vi "Tote Barrel Array Test.vi"() -> ()   [LabVIEW 2014]
panel:
  in  "Release":bool
  in  "Height":dbl
  out "Array Index":dbl
  out "Array Output":dbl
  in  "Down Button":bool
  in  "Up Button":bool
  in  "Grab Barrel":bool
  in  "Grab Tote":bool
  out "Barrel Grab":bool
  out "Tote Grabbed":bool
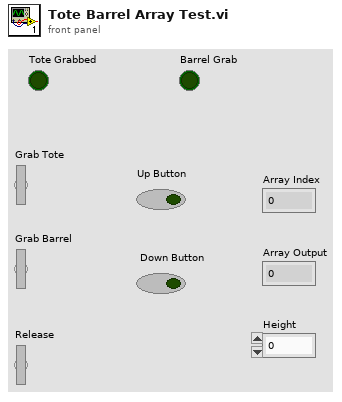
[diagram p1: front panel]
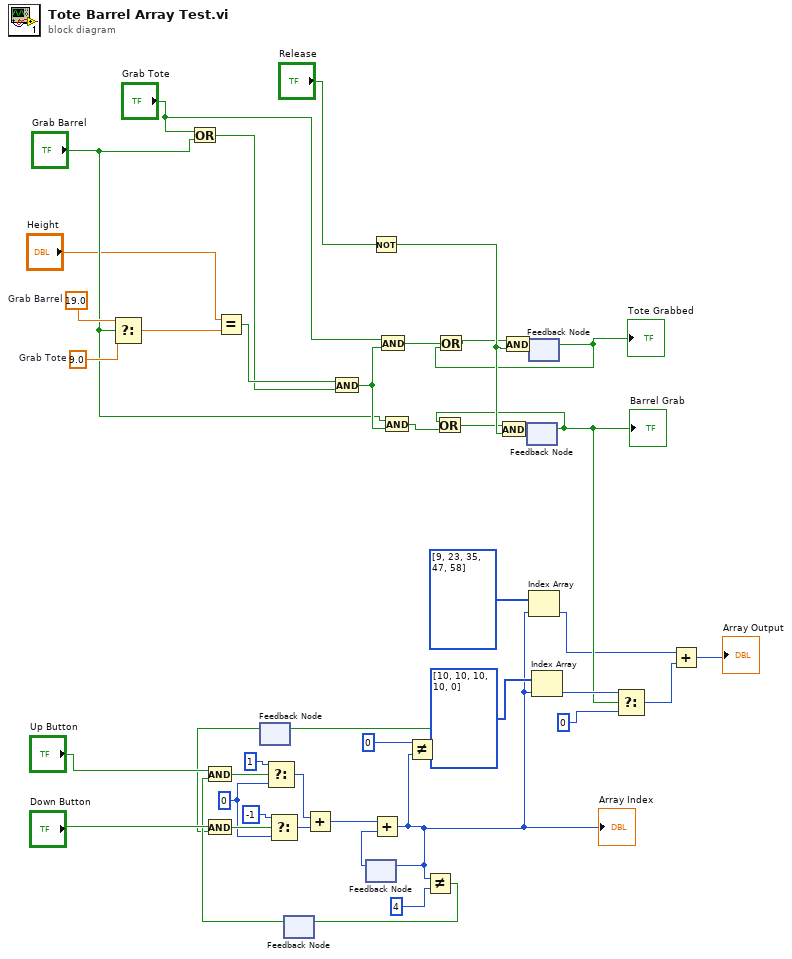
[diagram p0: block diagram]
diagram:
  w33 = 0
  w42 = 19.0  # Grab Barrel
  w43 = 9.0  # Grab Tote
  n1 = Select(t=w42, s="Grab Barrel", f=w43) -> (s? t:f=w41:dbl)
  n2 = Or(x="Grab Tote", y="Grab Barrel") -> (x .or. y?=w38:bool)
  n3 = Equal?(x="Height", y=w41) -> (x = y?=w44:bool)
  n4 = feedback #1() -> (w18:bool)  [unwired: 1 in]
  n5 = And(x="Down Button", y=w18) -> (x .and. y?=w37:bool)
  n6 = Select(t=-1, s=w37, f=w33) -> (s? t:f=w31:i32)
  n7 = feedback #2() -> (w21:bool)  [unwired: 1 in]
  n8 = And(x="Up Button", y=w21) -> (x .and. y?=w36:bool)
  n9 = Select(t=1, s=w36, f=w33) -> (s? t:f=w32:i32)
  n10 = Add(x=w32, y=w31) -> (x+y=w28:i32)
  n11 = And(x=w44, y=w38) -> (x .and. y?=w40:bool)
  n12 = feedback #3() -> (w15:i32)  [unwired: 1 in]
  n13 = Not(x="Release") -> (.not. x?=w8:bool)
  n14 = Add(x=w28, y=w15) -> (x+y=w14:i32)
  "Array Index" <- w14
  n15 = feedback-in #3(w14) -> ()
  n16 = And(x="Grab Tote", y=w40) -> (x .and. y?=w11:bool)
  n17 = And(x="Grab Barrel", y=w40) -> (x .and. y?=w10:bool)
  n18 = Not Equal?(x=0, y=w14) -> (x != y?=w19:bool)
  n19 = feedback-in #1(w19) -> ()
  n20 = Not Equal?(x=w14, y=4) -> (x != y?=w22:bool)
  n21 = feedback-in #2(w22) -> ()
  n22 = feedback #4() -> (w2:bool)  [unwired: 1 in]
  "Barrel Grab" <- w2
  n23 = Or(x=w2, y=w10) -> (x .or. y?=w7:bool)
  n24 = And(x=w7, y=w8) -> (x .and. y?=w3:bool)
  n25 = feedback-in #4(w3) -> ()
  n26 = feedback #5() -> (w4:bool)  [unwired: 1 in]
  "Tote Grabbed" <- w4
  n27 = Or(x=w11, y=w4) -> (x .or. y?=w6:bool)
  n28 = And(x=w6, y=w8) -> (x .and. y?=w5:bool)
  n29 = feedback-in #5(w5) -> ()
  n30 = Index Array(array=i32[] [9, 23, 35, 47, 58], index=w14) -> (element=w1:i32)
  n31 = Index Array(array=i32[] [10, 10, 10, 10, 0], index=w14) -> (element=w27:i32)
  n32 = Select(t=w27, s=w2, f=0) -> (s? t:f=w24:i32)
  n33 = Add(x=w1, y=w24) -> (x+y=→"Array Output":i32)
